vi "Read_Measurements.vi"(8 "error in (no error)":errorcluster, 11 "BMP208 in":refnum<class "BMP208.lvclass">) -> (0 "error out":errorcluster, 2 "Measurements":T1, 3 "BMP208 out":refnum<class "BMP208.lvclass">)   [LabVIEW 2020, in "BMP208.lvclass"]
uses:
  BMP208.lvclass
  Controls/td_cluster_measurements.ctl
  BMP208.lvclass/BMP208.ctl
  Properties/Read TempCoeff.vi
  Properties/Read PressCoeff.vi
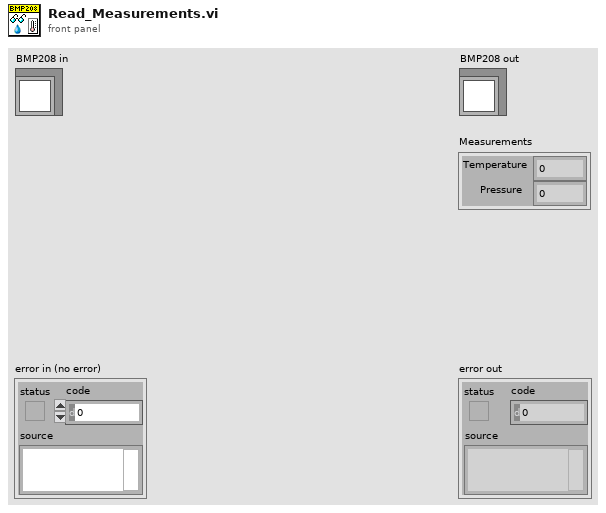
[diagram p1: front panel]
types:
  T1 = typedef "BMP208.lvclass/td_cluster_measurements.ctl" = cluster{"Temperature":dbl, "Pressure":dbl}
  T2 = typedef "BMP208.lvclass/td_cluster_Temp_Coeff.ctl" = cluster{"T1":u16, "T2":i16, "T3":i16}
  T3 = typedef "BMP208.lvclass/td_cluster_Press_Coeff.ctl" = cluster{"P1":u16, "P2":i16, "P3":i16, "P4":i16, "P5":i16, "P6":i16, "P7":i16, "P8":i16, "P9":i16}
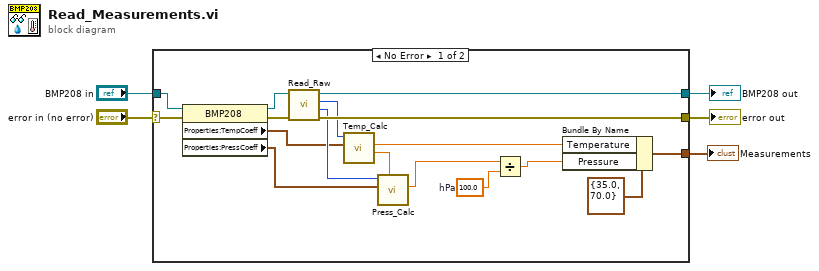
[diagram p0: block diagram]
diagram:
  n1 = case shown="No Error" "error in (no error)" {
    selector: "error in (no error)" -> [w19 w24]
    tunnel: [w16 w24] -> w4
    tunnel: [w14 w23] -> w2
    tunnel: "BMP208 in" -> [w17 w23]
    tunnel: [w21 _] -> w1
    frame No Error {
      w6 = 100.0  # hPa
      n2 = property class="BMP208"(reference=w17, error in=w19) -> (reference out=w15:refnum<class "BMP208.lvclass">, error out=w18:errorcluster, "Properties:TempCoeff"=w11:T2, "Properties:PressCoeff"=w10:T3)
      n3 = call "Read_Raw.vi"("error in (no error)"=w18, "BMP208 in"=w15) -> ("error out"=w16:errorcluster, "PressureU32"=w12:u32, "TempU32"=w13:u32, "BMP208 out"=w14:refnum<class "BMP208.lvclass">)  [unwired: 6 in]
      n4 = call "Temp_Calc.vi"("TempCoeff"=w11, "raw_temp"=w13) -> ("tfine"=w8:dbl, "Temperature"=w20:dbl)  [unwired: 8 in]
      n5 = call "Press_Calc.vi"("tfine"=w8, "PressCoeff"=w10, "PressureReadingU32"=w12) -> ("Pressure(Pa)"=w9:dbl)  [unwired: 8 in]
      n6 = Divide(x=w9, y=w6) -> (x/y=w7:dbl)
      n7 = Bundle By Name(cluster=T1 {"Temperature"=35.0, "Pressure"=70.0} ("Measurements"), "Temperature"=w20, "Pressure"=w7) -> (w21:T1)
    }
    frame Error {
    }
  }
  "error out" <- w4
  "BMP208 out" <- w2
  "Measurements" <- w1
